vi "flatten unflatten equality.vi"() -> ()   [LabVIEW 2017]
uses:
  Controls/dsf configuration file/1.0.0/dsf configuration.ctl
  Controls/dsf configuration file/1.0.0/version.ctl
  Controls/dsf configuration file/1.0.0/dsf plugin.ctl
  Controls/dsf configuration file/1.0.0/dsf timing.ctl
  Controls/dsf configuration file/1.0.0/dsf group.ctl
  Controls/dsf configuration file/1.0.0/dsf transfer.ctl
  Controls/dsf configuration file/1.0.0/dsf channel.ctl
  Controls/dsf configuration file/1.0.0/dsf settings.ctl
  DSF Configuration API v1.0.0.lvlib
  Controls/dsf configuration file/1.0.0/dsf configuration file v1.0.0.lvlib
panel:
  out "equal?":T1
  in  "configuration cluster in":T2
  # "dsf\nfile"
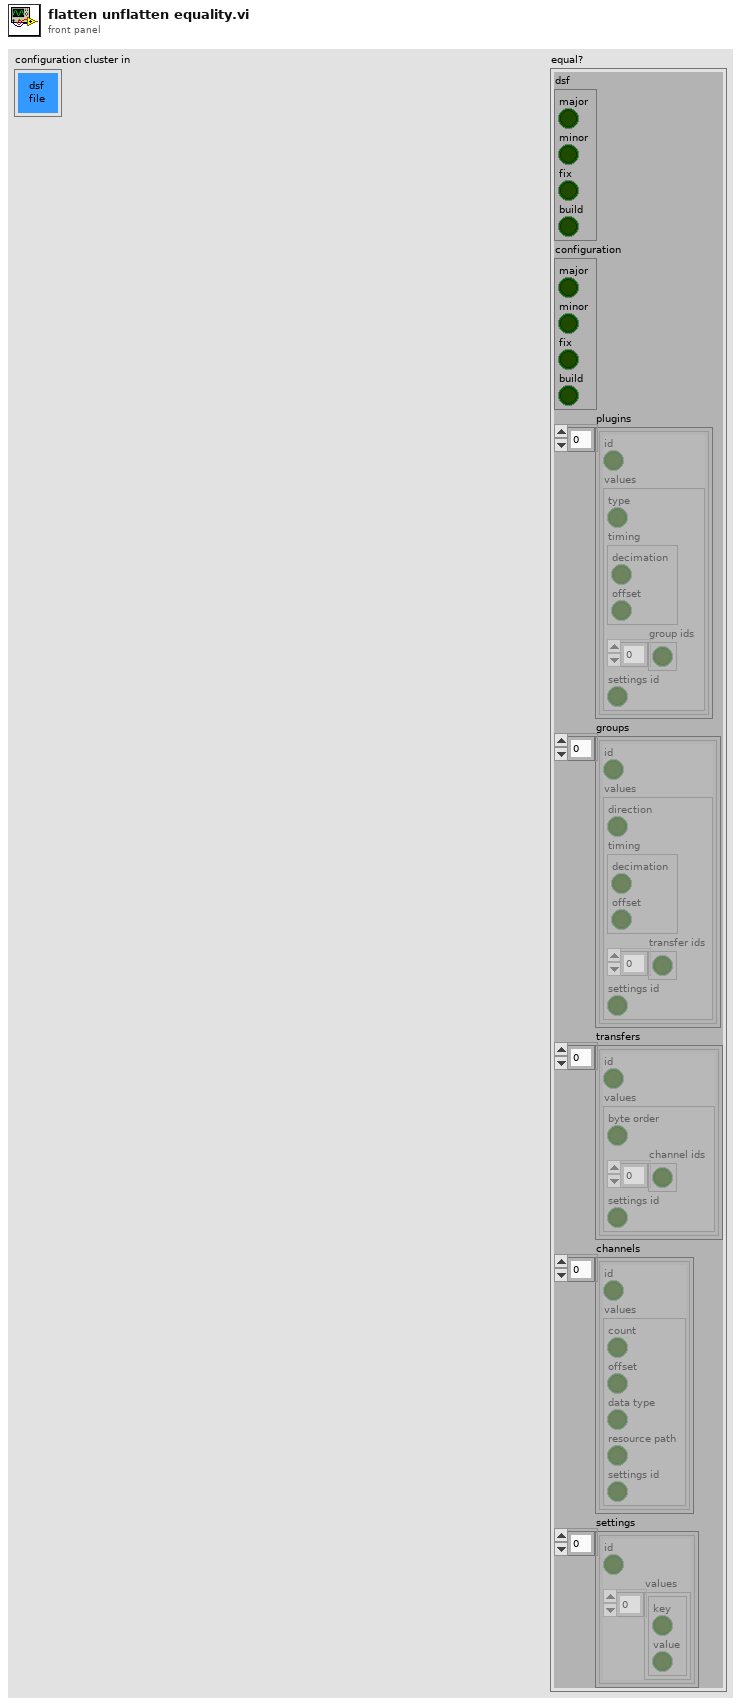
[diagram p1: front panel]
types:
  T1 = cluster{"dsf":cluster{"major":bool, "minor":bool, "fix":bool, "build":bool}, "configuration":cluster{"major":bool, "minor":bool, "fix":bool, "build":bool}, "plugins":cluster{"id":bool, "values":cluster{"type":bool, "timing":cluster{"decimation":bool, "offset":bool}, "group ids":bool[], "settings id":bool}}[], "groups":cluster{"id":bool, "values":cluster{"direction":bool, "timing":cluster{"decimation":bool, "offset":bool}, "transfer ids":bool[], "settings id":bool}}[], "transfers":cluster{"id":bool, "values":cluster{"byte order":bool, "channel ids":bool[], "settings id":bool}}[], "channels":cluster{"id":bool, "values":cluster{"count":bool, "offset":bool, "data type":bool, "resource path":bool, "settings id":bool}}[], "settings":cluster{"id":bool, "values":cluster{"key":bool, "value":bool}[]}[]}
  T2 = typedef "dsf configuration file v1.0.0.lvlib/dsf configuration.ctl" = cluster{"dsf":T3, "configuration":T3, "plugins":T4[], "groups":T6[], "transfers":T7[], "channels":T8[], "settings":T9[]}
  T3 = typedef "dsf configuration file v1.0.0.lvlib/version.ctl" = cluster{"major":u32, "minor":u32, "fix":u32, "build":string}
  T4 = typedef "dsf configuration file v1.0.0.lvlib/dsf plugin.ctl" = cluster{"id":string, "values":cluster{"type":string, "timing":T5, "group ids":string[], "settings id":string}}
  T5 = typedef "dsf configuration file v1.0.0.lvlib/dsf timing.ctl" = cluster{"decimation":i32, "offset":i32}
  T6 = typedef "dsf configuration file v1.0.0.lvlib/dsf group.ctl" = cluster{"id":string, "values":cluster{"direction":i32, "timing":T5, "transfer ids":string[], "settings id":string}}
  T7 = typedef "dsf configuration file v1.0.0.lvlib/dsf transfer.ctl" = cluster{"id":string, "values":cluster{"byte order":i32, "channel ids":string[], "settings id":string}}
  T8 = typedef "dsf configuration file v1.0.0.lvlib/dsf channel.ctl" = cluster{"id":string, "values":cluster{"count":i32, "offset":i32, "data type":i32, "resource path":string, "settings id":string}}
  T9 = typedef "dsf configuration file v1.0.0.lvlib/dsf settings.ctl" = cluster{"id":string, "values":cluster{"key":string, "value":string}[]}
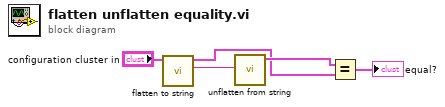
[diagram p0: block diagram]
diagram:
  n1 = call "flatten to string.vi"("configuration cluster in"="configuration cluster in") -> ("string"=w5:string, "configuration cluster out"=w2:T2)  [unwired: 8 in, 1 out]
  n2 = call "unflatten from string.vi"("String"=w5) -> ("dsf configuration out"=w3:T2)  [unwired: 9 in, 1 out]
  n3 = Equal?(x=w3, y=w2) -> (x = y?=→"equal?":T1)
